vi "get_pixel_rate.vi"(8 "error in (no error)":errorcluster, 11 "GenericTrajectory in":refnum<class "GenericTrajectory.lvclass">) -> (0 "error out":errorcluster, 1 "pixel dwell time":dbl[unit], 2 "pixel rate":dbl[unit], 3 "GenericTrajectory out":refnum<class "GenericTrajectory.lvclass">)   [LabVIEW 2010, in "GenericTrajectory.lvclass"]
doc: "returns the scanning rate in Hz (i.e., pixels per second) and the pixel dwell time"
uses:
  GenericTrajectory.lvclass
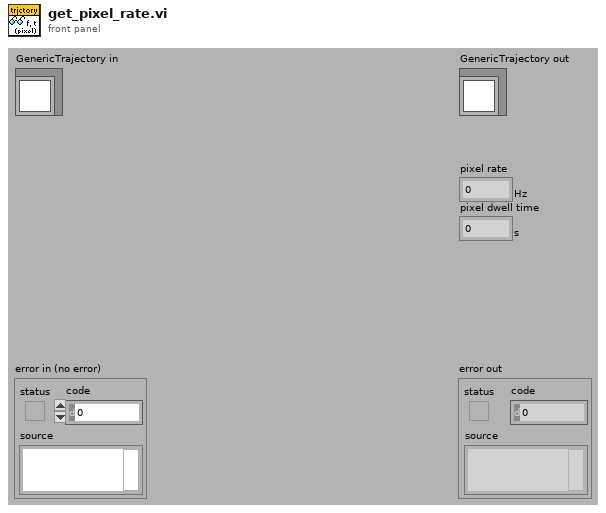
[diagram p1: front panel]
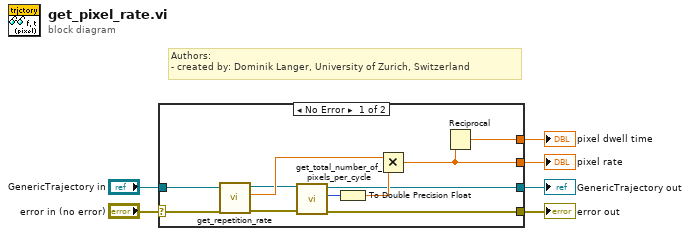
[diagram p0: block diagram]
diagram:
  # "Authors: \n- created by: Dominik Langer, University of Zurich, Switzerland"
  n1 = case shown="No Error" "error in (no error)" {
    selector: "error in (no error)" -> [w13 w19]
    tunnel: [w12 w19] -> w5
    tunnel: [w9 w18] -> w3
    tunnel: "GenericTrajectory in" -> [w10 w18]
    tunnel: [w8 _] -> w2
    tunnel: [w7 _] -> w1
    frame No Error {
      n2 = call-dynamic "get_repetition_rate.vi"("error in (no error)"=w13, "GenericTrajectory in"=w10) -> ("error out"=w14:errorcluster, "repetition rate"=w17:dbl[unit], "GenericTrajectory out"=w11:refnum<class "GenericTrajectory.lvclass">)  [unwired: 7 in]
      n3 = call-dynamic "get_total_number_of_pixels_per_cycle.vi"("error in (no error)"=w14, "GenericTrajectory in"=w11) -> ("error out"=w12:errorcluster, "total number of pixels per cycle"=w16:i32, "GenericTrajectory out"=w9:refnum<class "GenericTrajectory.lvclass">)  [unwired: 7 in]
      n4 = To Double Precision Float(number=w16) -> (double precision float=w15:dbl)
      n5 = Multiply(x=w17, y=w15) -> (x*y=w8:dbl[unit])
      n6 = Reciprocal(x=w8) -> (1/x=w7:dbl[unit])
    }
    frame Error {
    }
  }
  "error out" <- w5
  "GenericTrajectory out" <- w3
  "pixel rate" <- w2
  "pixel dwell time" <- w1
